vi "Attenuator_Communication.vi"(2 "错误输入":errorcluster) -> (0 "错误输出":errorcluster, 1 "通信成功？":bool)   [LabVIEW 2018]
panel:
  out "function return 2":i32
  out "function return":i32
  # "使用USB的驱动器"
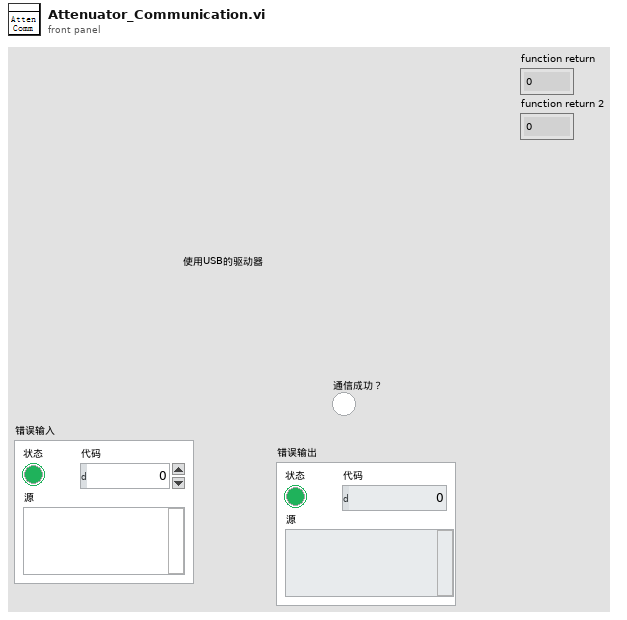
[diagram p1: front panel]
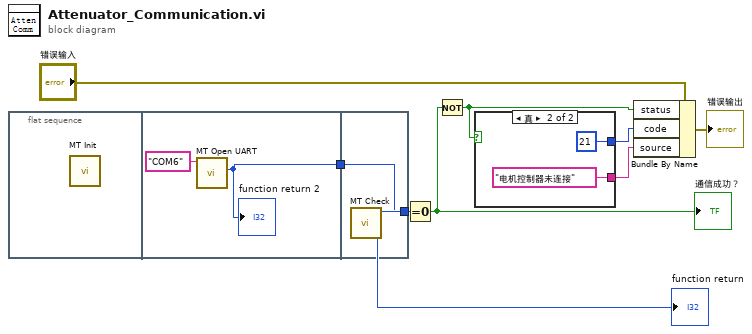
[diagram p0: block diagram]
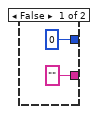
[diagram p2: hidden frame]
diagram:
  n1 = flat-sequence {
    tunnel: [w10] -> w1
    tunnel: [w11] -> w2
    tunnel: w1 -> [w11]
    frame #0 {
      n2 = call "MT Init.vi"() -> ()  [unwired: 10 in, 2 out]
    }
    frame #1 {
      n3 = call "MT Open UART.vi"("sCOM"="COM6") -> ("function return"=w10:i32)  [unwired: 8 in, 2 out]
      "function return 2" <- w10
    }
    frame #2 {
      n4 = call "MT Check.vi"() -> ()  [unwired: 10 in, 2 out]
    }
  }
  n5 = Equal To 0?(x=w2) -> (x = 0?=w4:bool)
  "通信成功？" <- w4
  n6 = Not(x=w4) -> (.not. x?=w8:bool)
  n7 = case shown="真" w8 {
    tunnel: ["" "电机控制器未连接" ("source")] -> w7
    tunnel: [0 ("code") 21 ("code")] -> w5
    frame False {
    }
    frame True {
    }
  }
  n8 = Bundle By Name(cluster="错误输入", "status"=w8, "code"=w5, "source"=w7) -> (→"错误输出":errorcluster)
  "function return" <- w2
